vi "checkIfconnected.vi"(7 "input stream cluster":T2, 8 "input error":errorcluster, 9 "Input device state":T1) -> (0 "error out":errorcluster, 1 "NextDeviceState":T1, 2 "Connected":bool)   [LabVIEW 2018]
uses:
  support/Network Stream Writer.ctl
  NetworkStream/NetworkStreamData.ctl
  Tektronik3102/Tecktronik action loop.ctl
  <resource>/objmgr/ni.dex.rc
  NetworkStream/NetworkStream.lvlib
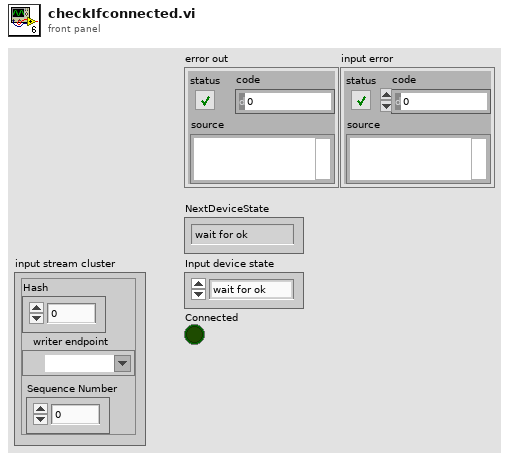
[diagram p1: front panel]
types:
  T1 = typedef "Tecktronik action loop.ctl" = enum16{"wait for ok", "error", "ready", "write log file", "waiting for connection", "exit", "sending command"}
  T2 = typedef "Network Stream Writer.ctl" = cluster{"Hash":u64, "writer endpoint":refnum<k21>, "Sequence Number":u64}
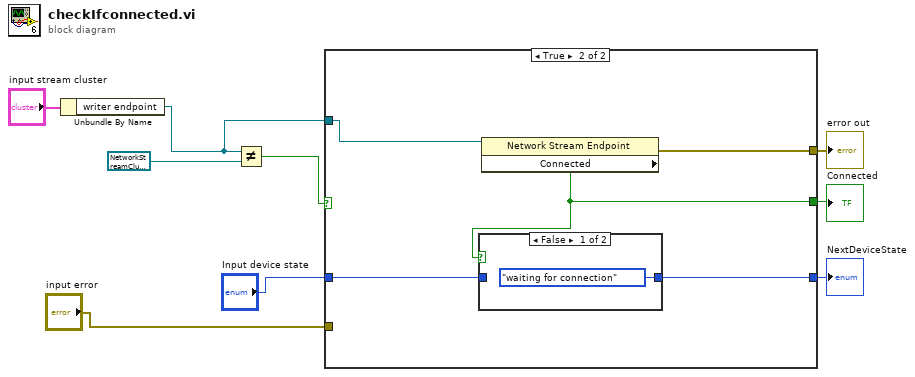
[diagram p0: block diagram]
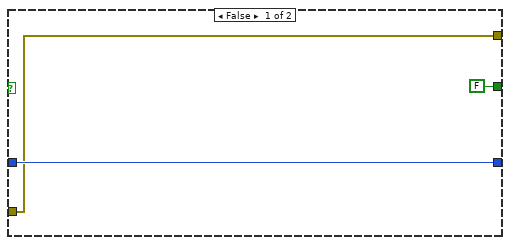
[diagram p2: hidden frame]
diagram:
  n1 = Unbundle By Name("input stream cluster") -> ("writer endpoint"=w6:refnum<k21>)
  n2 = Not Equal?(x=w6, y=refnum<k21> refnum ("writer endpoint")) -> (x != y?=w7:bool)
  n3 = case shown="True" w7 {
    tunnel: w6 -> [_ w17]
    tunnel: [w12 w16] -> w5
    tunnel: "Input device state" -> [w12 w15]
    tunnel: [w11 w14] -> w3
    tunnel: "input error" -> [w11 _]
    tunnel: [FALSE ("Connected") w13] -> w1
    frame False {
    }
    frame True {
      n4 = property class="Network Stream Endpoint"(reference=w17) -> (error out=w14:errorcluster, "Connected"=w13:bool)  [unwired: 1 in, 1 out]
      n5 = case shown="False" w13 {
        tunnel: [Tecktronik_action_loop."waiting for connection" ("DeviceState") w19] -> w16
        tunnel: w15 -> [_ w19]
        frame False {
        }
        frame True {
        }
      }
    }
  }
  "NextDeviceState" <- w5
  "error out" <- w3
  "Connected" <- w1
